vi "Configure Frequency.vi"   [LabVIEW 2023, in "Anritsu Signal Analyzer Series.lvlib"]
doc: "Configures Frequency settings."
uses:
  Anritsu Signal Analyzer Series.lvlib
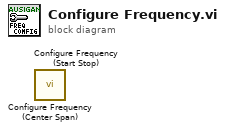
[diagram p0: block diagram]
diagram:
  n1 = call "Configure Frequency (Center Span).vi"() -> ()  [unwired: 14 in, 2 out]
  n2 = call "Configure Frequency (Start Stop).vi"() -> ()  [unwired: 14 in, 2 out]
